vi "Control solonoids in periodic tasks, shift registers.vi"(8 "Past Input Upper":bool, 11 "Past Input Closer":bool) -> (0 "New Input Upper":bool, 3 "New Input Closer":bool)   [LabVIEW 2017]
uses:
  <vilib>/Rock Robotics/WPI/Solenoid/WPI_SolenoidValue.ctl
  Robot Global Data.vi
  <vilib>/Rock Robotics/WPI/Solenoid/WPI_SolenoidSetEnum.vi
panel:
  # "To be placed in a loop with shift registers"
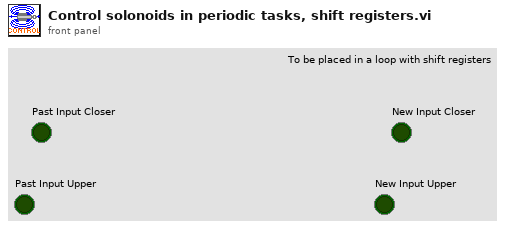
[diagram p1: front panel]
types:
  T1 = typedef "WPI_SolenoidValue.ctl" = enum16{"Off", "On", "Forward", "Reverse"}
  T2 = typedef "WPI_SolenoidDevRef.ctl" = cluster{"DevStatus":errorcluster, "Pneumatics Control Module":u8, "Forward Solenoid Channel":T3, "Reverse Solenoid Channel":T3}
  T3 = typedef "WPI_SolenoidChannel.ctl" = enum8{"Solenoid 0", "Solenoid 1", "Solenoid 2", "Solenoid 3", "Solenoid 4", "Solenoid 5", "Solenoid 6", "Solenoid 7", "Invalid"}
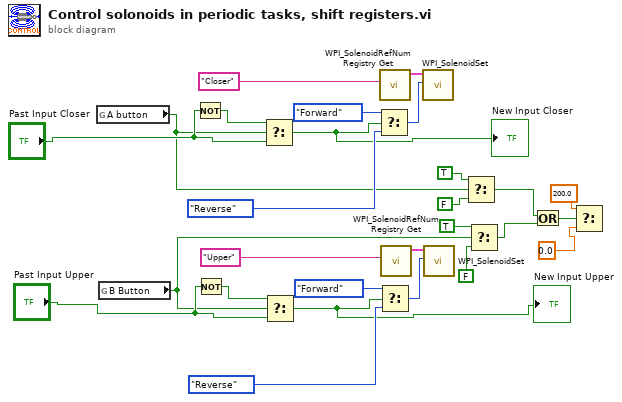
[diagram p0: block diagram]
diagram:
  n1 = global read "Robot Global Data.vi" "A button"() -> (w11:bool)
  n2 = global read "Robot Global Data.vi" "B Button"() -> (w10:bool)
  n3 = Not(x="Past Input Closer") -> (.not. x?=w21:bool)
  n4 = Not(x="Past Input Upper") -> (.not. x?=w22:bool)
  n5 = Select(t=w21, s=w11, f="Past Input Closer") -> (s? t:f=w15:bool)
  "New Input Closer" <- w15
  n6 = Select(t=w22, s=w10, f="Past Input Upper") -> (s? t:f=w12:bool)
  "New Input Upper" <- w12
  n7 = Select(t=WPI_SolenoidValue."Forward" ("Value"), s=w15, f=WPI_SolenoidValue."Reverse" ("Value")) -> (s? t:f=w20:T1)
  n8 = call <vilib>:"WPI_SolenoidRefNum Registry Get.vi"("refnum name"="Closer") -> ("SolenoidDevRef"=w17:T2)  [unwired: 9 in, 1 out]
  n9 = Select(t=WPI_SolenoidValue."Forward" ("Value"), s=w12, f=WPI_SolenoidValue."Reverse" ("Value")) -> (s? t:f=w23:T1)
  n10 = call <vilib>:"WPI_SolenoidRefNum Registry Get.vi"("refnum name"="Upper") -> ("SolenoidDevRef"=w26:T2)  [unwired: 9 in, 1 out]
  n11 = call-poly <vilib>:"WPI_SolenoidSet.vi"("Value"=w20, "SolenoidDevRef"=w17) -> ()  [unwired: 8 in, 2 out]
  n12 = call-poly <vilib>:"WPI_SolenoidSet.vi"("Value"=w23, "SolenoidDevRef"=w26) -> ()  [unwired: 8 in, 2 out]
  n13 = Select(t=TRUE, s=w11, f=FALSE) -> (s? t:f=w9:bool)
  n14 = Select(t=TRUE, s=w10, f=FALSE) -> (s? t:f=w8:bool)
  n15 = Or(x=w9, y=w8) -> (x .or. y?=w4:bool)
  n16 = Select(t=200.0, s=w4, f=0.0) -> ()  [unwired: 1 out]
